vi "Ophir_check.vi"() -> ()   [LabVIEW 2018]
panel:
  out "Ready Status":bool
  in  "System Stop":bool
  in  "Tab Control":T1(tab)
  in  "Ophir 2 Info":u16(ring)=1 caption="Info" items=["Device : JUNO; s/n:903794", "Head : PD300-IRG-v1; s/n:908004"]
  out "Ophir 2 Initialization":bool caption="Initialization"
  out "Ophir 2 MAX":dbl caption="MAX" format="%#_5g"
  in  "Ophir 2 Clear":bool caption="Clear"
  out "Ophir 2 Optical Power":dbl caption="Power" format="%#_4g"
  in  "Ophir 2 units":string(combo)="1000" caption="Units"
  in  "Ophir 2 Wait":u32=100 caption="Wait"
  out "Ophir 2 Over Range":bool caption="Over Range"
  out "Ophir 2 Char":dbl(graph)=6.67426339573744e-05
  in  "Ophir Select Communication Protocol":u16(ring) caption="Select Communication Protocol" items=["USB", "RS232", "GPIB"]
  in  "Ophir usb channel":i16 caption="usb channel"
  in  "Ophir Port Number (2)":i16=2 caption="Port Number (default 2)" min=0 max=20
  in  "Ophir Baud Rate (3:9600)":i16(ring)=3 caption="Baud Rate (3:9600)" items=["300", "1200", "4800", "9600", "19200", "38400"]
  in  "Ophir GPIB Address (10)":string="10" caption="GPIB Address (10)"
  out "Ophir 2 dup Visa Session":refnum<visa-resource-name>="USB0::0x0BD3::0x0777::NI-VISA-10003::RAW" caption="dup Visa Session"
  out "Ophir 2 Real Optical Power":dbl format="%.6e"
  out "Ophir 2 error out":errorcluster caption="error out"
  in  "Ophir error in (no error)":errorcluster caption="error in (no error)"
  out "Ophir 2 Status":bool caption="Ophir 2"
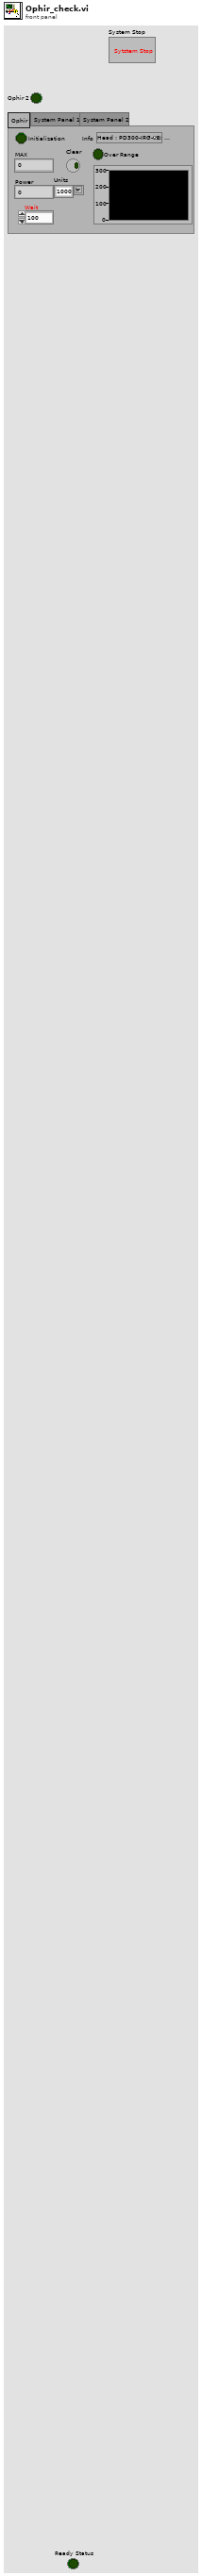
[diagram p1: front panel]
types:
  T1 = enum32{"Ophir", "System Panel 1", "System Panel 2"}
  T2 = enum8{"Enabled", "Disabled", "Disabled and Grayed Out"}
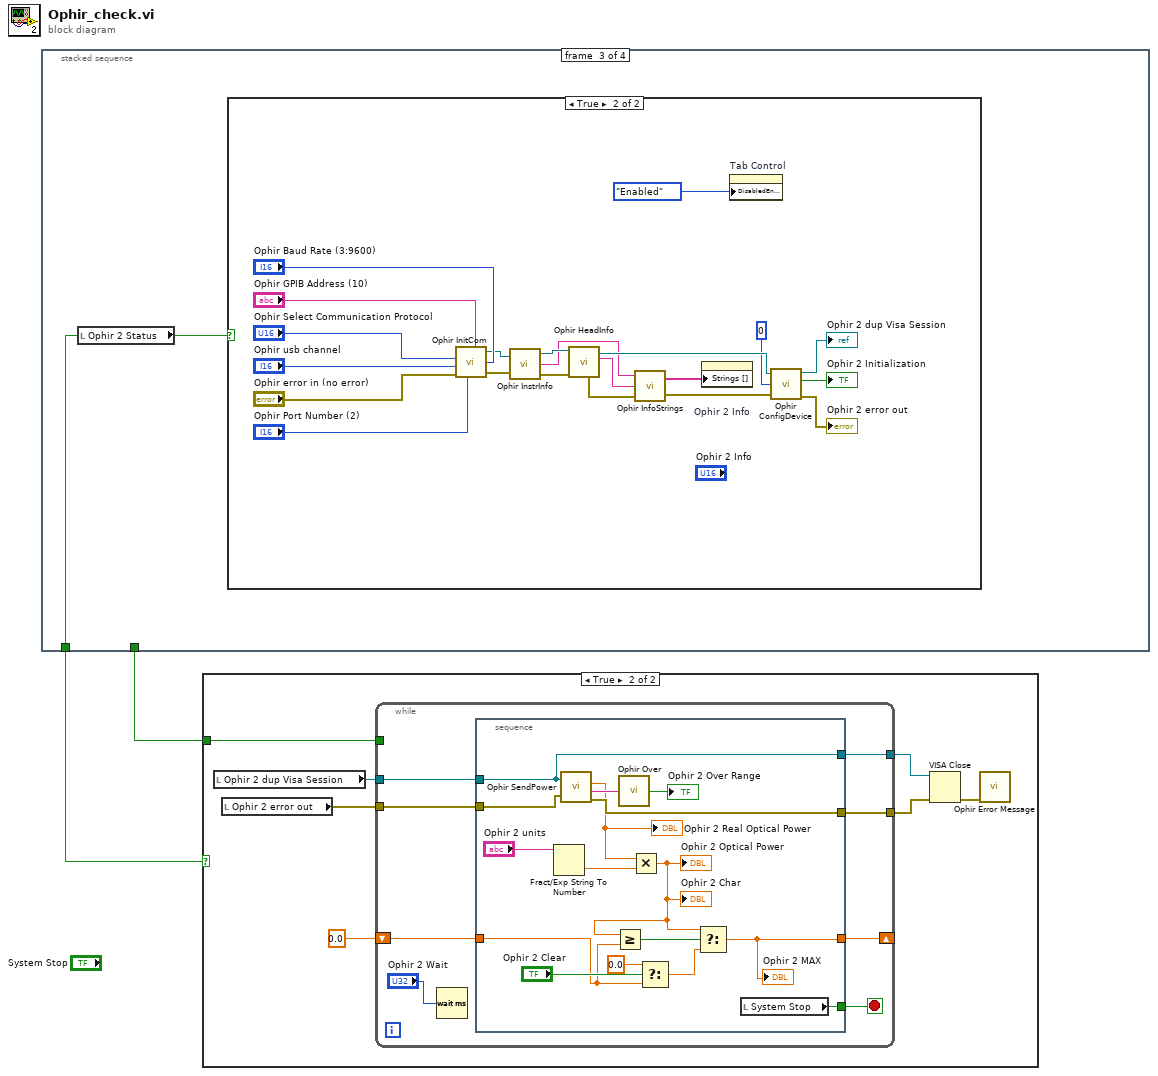
[diagram p0: block diagram]
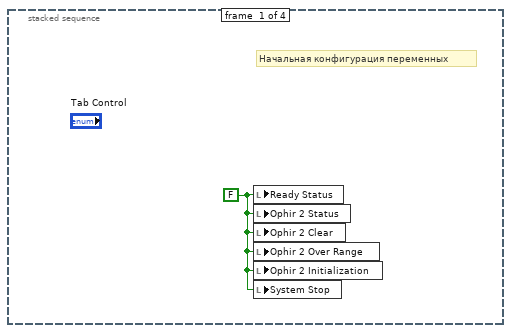
[diagram p2: hidden frame]
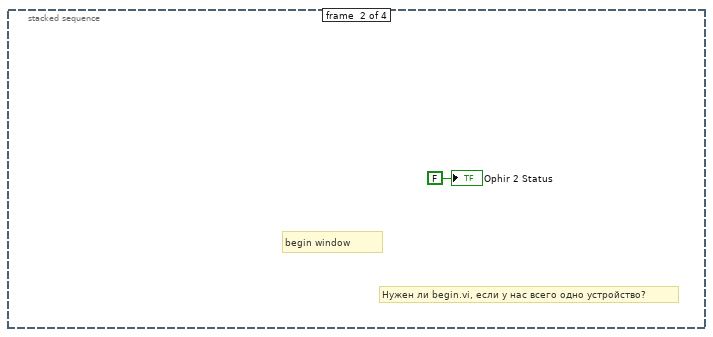
[diagram p3: hidden frame]
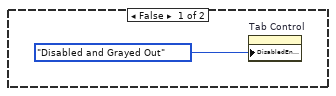
[diagram p4: hidden frame]
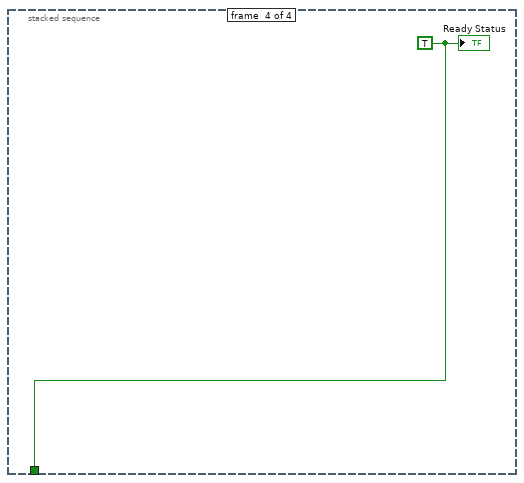
[diagram p5: hidden frame]
diagram:
  n1 = stacked-sequence {
    tunnel: [_ _ w5 _] -> w2
    tunnel: [_ _ _ w28] -> w1
    frame #0 {
      w3 = FALSE ("Ready Status")
      # "Начальная конфигурация переменных"
      n2 = local write "Ready Status"(w3) -> ()
      n3 = local write "Ophir 2 Status"(w3) -> ()
      n4 = local write "Ophir 2 Clear"(w3) -> ()
      n5 = local write "Ophir 2 Over Range"(w3) -> ()
      n6 = local write "Ophir 2 Initialization"(w3) -> ()
      n7 = local write "System Stop"(w3) -> ()
    }
    frame #1 {
      # "Нужен ли begin.vi, если у нас всего одно устройство?"
      # "begin window"
      "Ophir 2 Status" <- FALSE ("Ophir 2 Status")
    }
    frame #2 {
      n8 = local read "Ophir 2 Status"() -> (w5:bool)
      n9 = case shown="True" w5 {
        frame False {
          n10 = property on="Tab Control" class="TabCtl (strict)"("DisabledEnum"=T2."Disabled and Grayed Out" ("Disabled")) -> ()  [unwired: 2 in, 2 out]
        }
        frame True {
          n11 = call "Ophir InitCom.vi"("GPIB Address (default 10)"="Ophir GPIB Address (10)", "Communication (default USB 0)"="Ophir Select Communication Protocol", "USB Channel number (default 0)"="Ophir usb channel", "Port Number (default 2)"="Ophir Port Number (2)", "error in (no error)"="Ophir error in (no error)", "Baud Rate (3:9600)"="Ophir Baud Rate (3:9600)") -> ("dup Visa Session"=w13:refnum<visa-resource-name>, "error out"=w12:errorcluster)  [unwired: 1 out]
          n12 = call "Ophir InstrInfo.vi"("Visa Session"=w13, "error in (no error)"=w12) -> ("dup Visa Session"=w26:refnum<visa-resource-name>, "Instrument Info"=w22:string, "error out"=w24:errorcluster)
          n13 = call "Ophir HeadInfo.vi"("Visa Session"=w26, "error in (no error)"=w24) -> ("error out"=w23:errorcluster, "dup Visa Session"=w25:refnum<visa-resource-name>, "Head Info"=w21:string)  [unwired: 6 out]
          n14 = call "Ophir InfoStrings.vi"("error in (no error)"=w23, "Head Info"=w21, "Instrument Info"=w22) -> ("error out"=w20:errorcluster, "Strings Array"=w19:string[])
          n15 = property on="Ophir 2 Info" class="Ring (strict)"("Strings []"=w19) -> ()  [unwired: 2 in, 2 out]
          n16 = property on="Tab Control" class="TabCtl (strict)"("DisabledEnum"=T2."Enabled" ("Disabled")) -> ()  [unwired: 2 in, 2 out]
          n17 = call "Ophir ConfigDevice.vi"("Visa Session"=w25, "Measure Choice (0:Power)"=u16 0, "error in (no error)"=w20) -> ("dup Visa Session"=→"Ophir 2 dup Visa Session":refnum<visa-resource-name>, "OK ?"=→"Ophir 2 Initialization":bool, "error out"=→"Ophir 2 error out":errorcluster)  [unwired: 1 out]
        }
      }
    }
    frame #3 {
      w28 = TRUE ("Boolean")
      "Ready Status" <- w28
    }
  }
  n18 = case shown="True" w2 {
    tunnel: w1 -> [_ w30]
    frame False {
    }
    frame True {
      n19 = local read "Ophir 2 dup Visa Session"() -> (w32:refnum<visa-resource-name>)
      n20 = local read "Ophir 2 error out"() -> (w31:errorcluster)
      n21 = while {
        tunnel: [w43] -> w34
        tunnel: [w37] -> w33
        tunnel: w32 -> [w41]
        tunnel: w31 -> [w40]
        tunnel: w30 -> [_]
        shift-right: [w38] -> _
        shift-left: 0.0 -> [w39]
        stop <- w42 stop-if-true
        n22 = Wait (ms)(milliseconds to wait="Ophir 2 Wait") -> ()  [unwired: 1 out]
        n23 = stacked-sequence {
          tunnel: [w59] -> w43
          tunnel: [w44] -> w42
          tunnel: w41 -> [w45]
          tunnel: w40 -> [w54]
          tunnel: w39 -> [w48]
          tunnel: [w46] -> w38
          tunnel: [w45] -> w37
          frame #0 {
            n24 = Fract/Exp String To Number(string="Ophir 2 units") -> (number=w47:dbl)  [unwired: 3 in, 1 out]
            n25 = call "Ophir SendPower.vi"("Visa Session"=w45, "error in (no error)"=w54) -> ("Value Number"=w56:dbl, "Value String"=w57:string, "error out"=w59:errorcluster)  [unwired: 1 out]
            "Ophir 2 Real Optical Power" <- w56
            n26 = call "Ophir Over.vi"("Value String"=w57) -> ("Overrange"=→"Ophir 2 Over Range":bool)
            n27 = Multiply(x=w56, y=w47) -> (x*y=w52:dbl)
            "Ophir 2 Char" <- w52
            "Ophir 2 Optical Power" <- w52
            n28 = Greater Or Equal?(x=w52, y=w48) -> (x >= y?=w53:bool)
            n29 = Select(t=0.0, s="Ophir 2 Clear", f=w48) -> (s? t:f=w51:dbl)
            n30 = Select(t=w52, s=w53, f=w51) -> (s? t:f=w46:dbl)
            "Ophir 2 MAX" <- w46
            n31 = local read "System Stop"() -> (w44:bool)
          }
        }
      }
      n32 = VISA Close(VISA resource name=w33, error in (no error)=w34) -> (error out=w35:errorcluster)
      n33 = call "Ophir Error Message.vi"("error in (no error)"=w35) -> ()  [unwired: 3 in, 4 out]
    }
  }
